vi "NotWiredMessageSubVI.vi"(9 "Boolean Text.Text 2":string, 10 "Boolean Text.Text":string, 11 "Text.Text":string) -> (3 "cancel?":bool)   [LabVIEW 2017]
panel:
  in  "Label":string
  in  "Configure now":bool
  in  "Configure later":bool
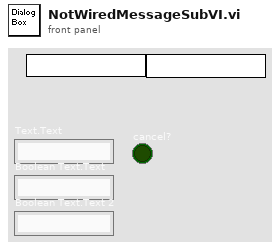
[diagram p1: front panel]
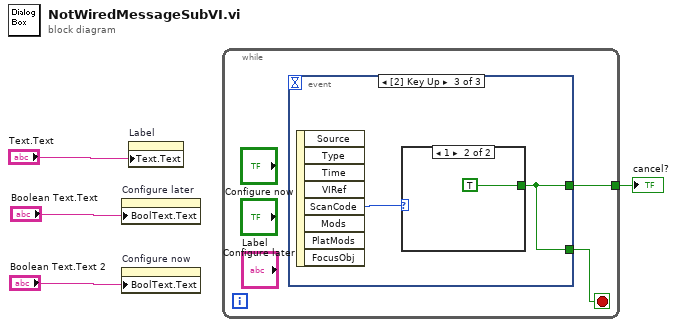
[diagram p0: block diagram]
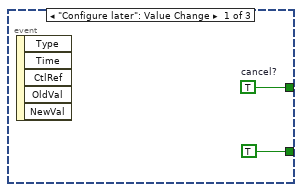
[diagram p2: hidden frame]
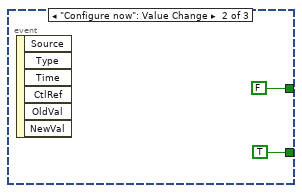
[diagram p3: hidden frame]
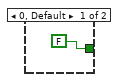
[diagram p4: hidden frame]
diagram:
  n1 = property on="Configure later" class="Bool"("BoolText.Text"="Boolean Text.Text") -> ()  [unwired: 2 in, 2 out]
  n2 = property on="Configure now" class="Bool"("BoolText.Text"="Boolean Text.Text 2") -> ()  [unwired: 2 in, 2 out]
  n3 = property on="Label" class="Str"("Text.Text"="Text.Text") -> ()  [unwired: 2 in, 2 out]
  n4 = while {
    tunnel: [w5] -> w4
    stop <- w6 stop-if-true
    n5 = event shown="[2] Key Up" {
      selector: _ -> [_ _ _]
      dyn-events: _ -> [_ _ _]
      timeout: _ -> [_ _ _]
      tunnel: [TRUE TRUE ("cancel?") w11] -> w6
      tunnel: [w7 FALSE ("cancel?") w11] -> w5
      event "Configure later": Value Change {
        w7 = TRUE  # cancel?
        n6 = event-data() -> ()  [unwired: 1 in, 5 out]
      }
      event "Configure now": Value Change {
        n7 = event-data() -> ()  [unwired: 1 in, 6 out]
      }
      event Key Up {
        n8 = event-data() -> ("ScanCode"=w12:i16)  [unwired: 1 in, 7 out]
        n9 = case shown="1" w12 {
          tunnel: [FALSE TRUE] -> w11
          frame 0, Default {
          }
          frame 1 {
          }
        }
      }
    }
  }
  "cancel?" <- w4
